vi "BatteryIndicator.vi"(10 "Numeric":dbl) -> ()   [LabVIEW 2021]
panel:
  out "Meter":dbl(knob)=21.586596923816817 scale=0.0..100.0
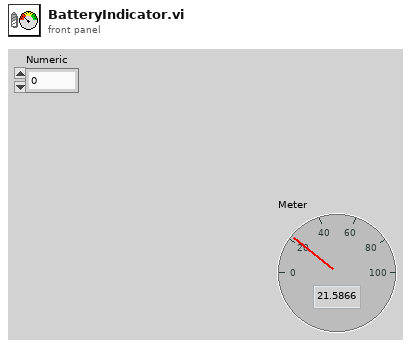
[diagram p1: front panel]
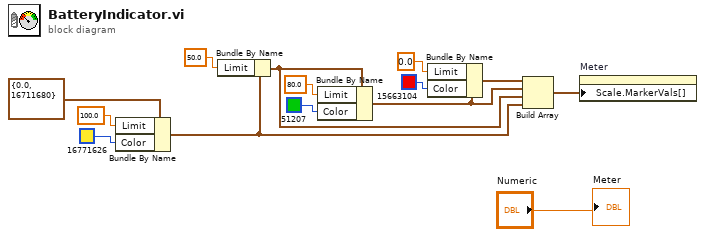
[diagram p0: block diagram]
diagram:
  n1 = Bundle By Name(cluster=cluster{"Limit":dbl, "Color":u32} {"Limit"=0.0, "Color"=16711680}, "Limit"=100.0 ("Limit 4"), "Color"=u32 16771626 ("Color 3")) -> (w8:cluster{"Limit":dbl, "Color":u32})
  n2 = Bundle By Name(cluster=w8, "Limit"=50.0 ("Limit 3")) -> (w9:cluster{"Limit":dbl, "Color":u32})
  n3 = Bundle By Name(cluster=w9, "Limit"=80.0 ("Limit 2"), "Color"=u32 51207 ("Color 2")) -> (w10:cluster{"Limit":dbl, "Color":u32})
  n4 = Bundle By Name(cluster=w10, "Limit"=0.0 ("Limit 1"), "Color"=u32 15663104 ("Color 1")) -> (w11:cluster{"Limit":dbl, "Color":u32})
  n5 = Build Array(w11, w10, w9, w8) -> (w7:cluster{"Limit":dbl, "Color":u32}[])
  n6 = property on="Meter" class="Knob (strict)"("Scale.MarkerVals[]"=w7) -> ()  [unwired: 2 in, 2 out]
  "Meter" <- "Numeric"
